vi "Mcp2210 Set Access Control.vi"(7 "accessConfig":u8(ring) items=["No Protection"=0, "Protected"=64, "Password Change"=165], 8 "error in (no error)":errorcluster, 9 "newPasswd":string, 10 "currentPasswd":string, 11 "handle":u32) -> (0 "error out":errorcluster, 1 "newPasswd out":string, 2 "currentPasswd out":string, 3 "handle out":u32)   [LabVIEW 2015, in "mcp2210.lvlib"]
doc: "Configures the NVRAM password protection.\nThe function returns 0 (E_SUCCESS) if the new access control configuration is accepted\nor negative error code in case of device communication failure or if the access control configuration\nchange is not accepted by the device.\nError codes in case of rejected configuration change:\n- E_ERR_NVRAM_LOCKED - NVRAM is permanently locked, no access control change is accepted\n- E_ERR_WRONG_PASSWD - old password mismatch, but the number of attempts is less than 5\n- E_ERR_ACCESS_DENIED - old password mismatch, but the number of attempts exceeded 5,\nso the NVRAM writes are blocked until the next device reset\n!!! Important notes !!!\n1. The password strings must have exactly 8 characters.\nIf they have a different number of characters, -2 (E_ERR_INVALID_PARAMETER) error code is returned.\n2. The new password string becomes effective after the next chip reset or power cycle. Therefore,\nif maximum protection is required, a chip reset is recommended after calling Mcp2210_SetAccessControl()\nwith accessConfig parameter set to MCP2210_NVRAM_PROTECTED or MCP2210_NVRAM_PASSWD_CHANGE.\nThe chip reset can be achieved using Mcp2210_Reset() API.\nParameters:\nInputs:\n- void *handle - The pointer to the USB device handle. Cannot be NULL.\n- unsigned char accessConfig\n- indicates which type of access control change is performed by the API call.\n- 0x0 (MCP2210_NVRAM_NO_PROTECTION) - disable the password protection:\nIf the password protection is enabled, the currentPassword must be\nvalid, otherwise the function returns negative error code:\nE_ERR_WRONG_PASSWD or E_ERR_ACCESS_DENIED\nIf the password protection is already disabled, the function\nignores the currentPassword and returns E_SUCCESS.\n- 0x40 (MCP2210_NVRAM_PROTECTED) - enable the password protection:\nIf the password protection is not enabled, newPassword must be a valid\npassword string.\nIf the password protection is already enabled, newPassword is ignored\nand the function returns negative error code: E_ERR_NVRAM_PROTECTED.\n- 0xA5 (MCP2210_NVRAM_PASSWD_CHANGE) - change the current password with\nthe new one if the password protection is already enabled.\nBoth currentPasswd and newPasswd must be valid password strings.\nIf the password protection is not enabled, the function returns\nnegative error code: E_ERR_PASSWD_CHANGE\n- char *currentPasswd - string of 8 characters (8 bytes), NULL terminated.\n- char *newPasswd - string of 8 characters (8 bytes), NULL terminated.\nOutputs:\n- none\nReturns:\n- 0 for success: E_SUCCESS\n- negative error code: E_ERR_NULL, E_ERR_INVALID_HANDLE_VALUE, E_ERR_INVALID_PARAMETER\nE_ERR_HID_TIMEOUT, E_ERR_HID_RW_FILEIO, E_ERR_UNKOWN_ERROR\nE_ERR_NVRAM_LOCKED, E_ERR_WRONG_PASSWD, E_ERR_ACCESS_DENIED\nE_ERR_NVRAM_PROTECTED, E_ERR_PASSWD_CHANGE\nE_ERR_CMD_ECHO, E_ERR_CMD_FAILED\n\nMCP2210_DLL_UM_API int __stdcall Mcp2210_SetAccessControl(void *handle, unsigned char accessConfig, char *currentPasswd, char *newPasswd);"
uses:
  <userlib>/mcp2210/mcp2210.lvlib
  <userlib>/mcp2210/mcp2210_dll_um_x86.dll
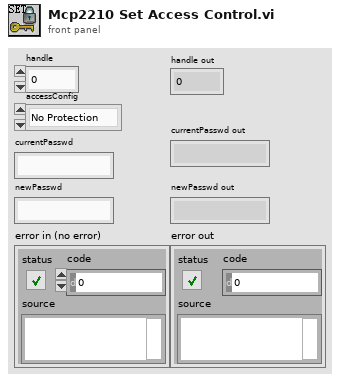
[diagram p1: front panel]
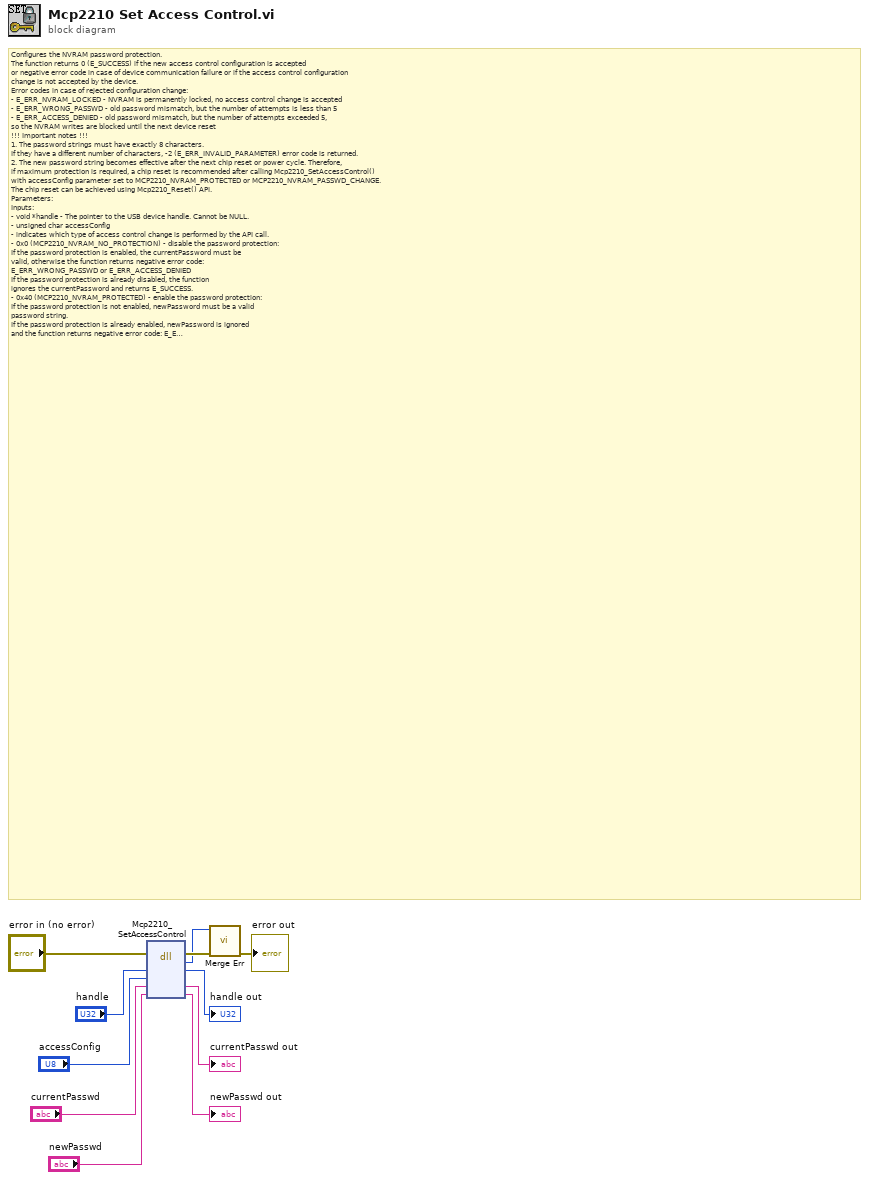
[diagram p0: block diagram]
diagram:
  # "Configures the NVRAM password protection.\nThe function returns 0 (E_SUCCESS) if the new access control configuration is accepted\nor negative error code in case of device communication failure or if the access control configuration\nchange is not accepted by the device.\nError codes in case of rejected configuration change:\n- E_ERR_NVRAM_LOCKED - NVRAM is permanently locked, no access control change is accepted\n- E_ERR_WRONG_PASSWD - old password mismatch, but the number of attempts is less than 5\n- E_ERR_ACCESS_DENIED - old password mismatch, but the number of attempts exceeded 5,\nso the NVRAM writes are blocked until the next device reset\n!!! Important notes !!!\n1. The password strings must have exactly 8 characters.\nIf they have a different number of characters, -2 (E_ERR_INVALID_PARAMETER) error code is returned.\n2. The new password string becomes effective after the next chip reset or power cycle. Therefore,\nif maximum protection is required, a chip reset is recommended after calling Mcp2210_SetAccessControl()\nwith accessConfig parameter set to MCP2210_NVRAM_PROTECTED or MCP2210_NVRAM_PASSWD_CHANGE.\nThe chip reset can be achieved using Mcp2210_Reset() API.\nParameters:\nInputs:\n- void *handle - The pointer to the USB device handle. Cannot be NULL.\n- unsigned char accessConfig\n- indicates which type of access control change is performed by the API call.\n- 0x0 (MCP2210_NVRAM_NO_PROTECTION) - disable the password protection:\nIf the password protection is enabled, the currentPassword must be\nvalid, otherwise the function returns negative error code:\nE_ERR_WRONG_PASSWD or E_ERR_ACCESS_DENIED\nIf the password protection is already disabled, the function\nignores the currentPassword and returns E_SUCCESS.\n- 0x40 (MCP2210_NVRAM_PROTECTED) - enable the password protection:\nIf the password protection is not enabled, newPassword must be a valid\npassword string.\nIf the password protection is already enabled, newPassword is ignored\nand the function returns negative error code: E_ERR_NVRAM_PROTECTED.\n- 0xA5 (MCP2210_NVRAM_PASSWD_CHANGE) - change the current password with\nthe new one if the password protection is already enabled.\nBoth currentPasswd and newPasswd must be valid password strings.\nIf the password protection is not enabled, the function returns\nnegative error code: E_ERR_PASSWD_CHANGE\n- char *currentPasswd - string of 8 characters (8 bytes), NULL terminated.\n- char *newPasswd - string of 8 characters (8 bytes), NULL terminated.\nOutputs:\n- none\nReturns:\n- 0 for success: E_SUCCESS\n- negative error code: E_ERR_NULL, E_ERR_INVALID_HANDLE_VALUE, E_ERR_INVALID_PARAMETER\nE_ERR_HID_TIMEOUT, E_ERR_HID_RW_FILEIO, E_ERR_UNKOWN_ERROR\nE_ERR_NVRAM_LOCKED, E_ERR_WRONG_PASSWD, E_ERR_ACCESS_DENIED\nE_ERR_NVRAM_PROTECTED, E_ERR_PASSWD_CHANGE\nE_ERR_CMD_ECHO, E_ERR_CMD_FAILED\n\nMCP2210_DLL_UM_API int __stdcall Mcp2210_SetAccessControl(void *handle, unsigned char accessConfig, char *currentPasswd, char *newPasswd);"
  n1 = dll-call lib="D:/LabVIEW 2015/user.lib/mcp2210/mcp2210_dll_um_x86.*" fn="Mcp2210_SetAccessControl"(error in="error in (no error)", "handle"="handle", "accessConfig"="accessConfig", "currentPasswd"="currentPasswd", "newPasswd"="newPasswd") -> (error out=w4:errorcluster, "return type"=w3:i32, "handle"=→"handle out":i32, "currentPasswd"=→"currentPasswd out":string, "newPasswd"=→"newPasswd out":string)  [unwired: 3 in, 1 out]
  n2 = call <userlib>:"Merge Err.vi"("error in (no error)"=w4, "return type"=w3) -> ("error out"=→"error out":errorcluster)  [unwired: 9 in]
